vi "TDTSyn-Close.vi"(0 "State in":T1, 11 "error in (no error)":errorcluster) -> (4 "State out":T1, 15 "error out":errorcluster)   [LabVIEW 2020]
uses:
  TDTSyn-State.ctl
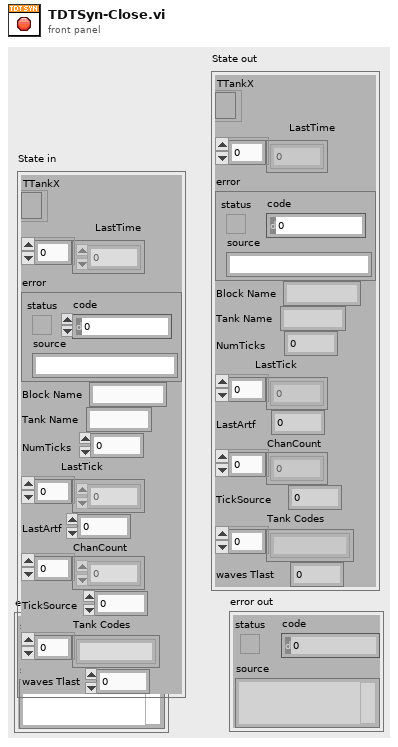
[diagram p1: front panel]
types:
  T1 = typedef "TDTSyn-State.ctl" = cluster{"TTankX":refnum<k7>, "LastTime":dbl[], "error":errorcluster, "Block Name":string, "Tank Name":string, "NumTicks":i32, "LastTick":dbl[], "LastArtf":dbl, "ChanCount":i32[], "TickSource":i32, "Tank Codes":string[], "waves Tlast":dbl}
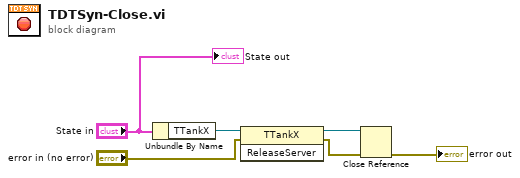
[diagram p0: block diagram]
diagram:
  n1 = Unbundle By Name("State in") -> ("TTankX"=w6:refnum<k7>)
  n2 = invoke class="TTankX" method="ReleaseServer"(reference=w6, error in="error in (no error)") -> (reference out=w5:refnum<k7>, error out=w4:errorcluster)  [unwired: 1 in, 1 out]
  n3 = Close Reference(reference=w5, error in (no error)=w4) -> (error out=→"error out":errorcluster)
  "State out" <- "State in"
